vi "Convert to Tree Cluster.vi"(8 "error in (no error)":errorcluster, 11 "Array in":T1[](array[typedef])) -> (0 "error out":errorcluster, 3 "Array out":T2[](array[typedef]))   [LabVIEW 2023, in "VIDoc Parsing.lvlib" / "Structure Reporter.lvlib"]
uses:
  Structure Reporter.lvlib
  Tree Cluster.ctl
  Structure Result 2.ctl
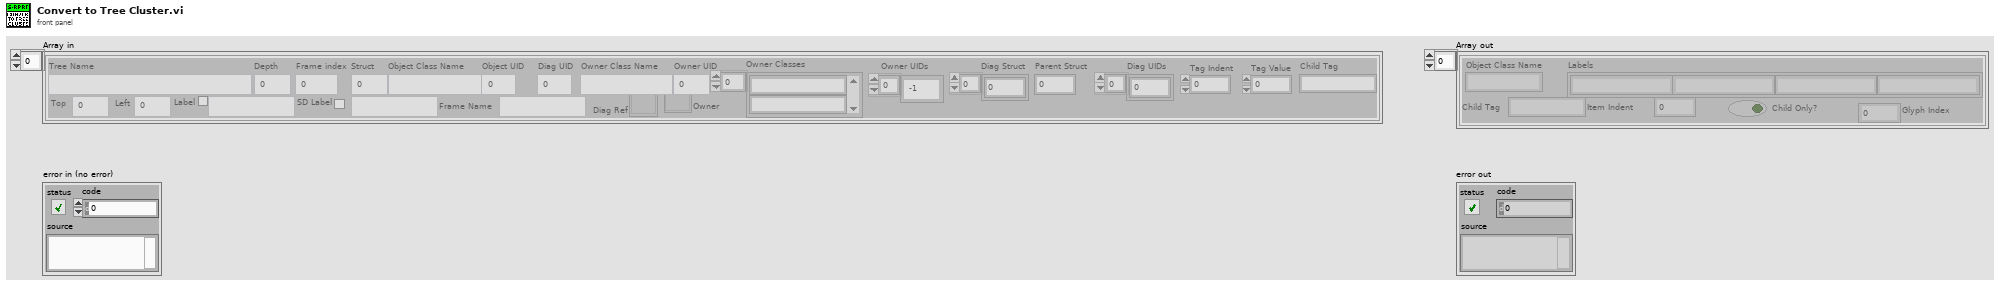
[diagram p1: front panel]
types:
  T1 = typedef "VIDoc Parsing.lvlib/Structure Reporter.lvlib/Structure Result 2.ctl" = cluster{"Depth":i32, "Top":i32, "Left":i32, "Frame index":i32, "Struct":i32, "Object Class Name":string, "Object UID":i32, "Label Visible":bool, "Object Label":string, "SD Label Visible":bool, "Object SD Label":string, "Frame Name":string, "Diag UID":i32, "Owner Class Name":string, "Owner UID":i32, "Diag Struct":i32[], "Parent Struct":i32, "Diag UIDs":i32[], "Tree Name":string, "Diag Ref":refnum<vi>, "Owner Classes":string[], "Owner":refnum<vi>, "Owner UIDs":i32[], "Tag Indent":i32, "Tag Value":i32, "Child Tag":string}
  T2 = typedef "VIDoc Parsing.lvlib/Structure Reporter.lvlib/Tree Cluster.ctl" = cluster{"Object Class Name":string, "Labels":string[], "Child Tag":string, "Item Indent":i32, "Child Only?":bool, "Glyph Index":i32}
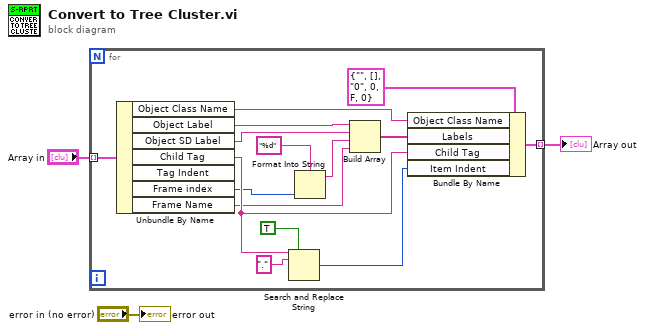
[diagram p0: block diagram]
diagram:
  n1 = for {
    tunnel: "Array in" -> [w17] mode=indexing
    tunnel: [w9] -> w3 mode=indexing
    n2 = Unbundle By Name(w17) -> ("Object Class Name"=w16:string, "Object Label"=w15:string, "Object SD Label"=w14:string, "Child Tag"=w12:string, "Frame index"=w5:i32, "Frame Name"=w4:string)  [unwired: 1 out]
    n3 = Search and Replace String(replace all?=TRUE ("replace all? (F)"), input string=w12, search string=".") -> (number of replacements=w10:i32)  [unwired: 5 in, 3 out]
    n4 = Format Into String(format string="%d", w5) -> (resulting string=w6:string)  [unwired: 2 in, 1 out]
    n5 = Build Array(w15, w14, w6, w4) -> (w13:string[])
    n6 = Bundle By Name(cluster=T2 {"Object Class Name"="", "Labels"=[], "Child Tag"="0", "Item Indent"=0, "Child Only?"=FALSE, "Glyph Index"=0} ("Item"), "Object Class Name"=w16, "Labels"=w13, "Child Tag"=w12, "Item Indent"=w10) -> (w9:T2)
  }
  "Array out" <- w3
  "error out" <- "error in (no error)"
